vi "ExpDetailsHeader.vi"(0 "error in (no error)":errorcluster) -> (1 "appended array":string[][](array[string]), 2 "error out":errorcluster)   [LabVIEW 2020]
panel:
  in  "OK Button":bool
  in  "Operator":string
  in  "Target's material":string
  in  "Experiment number":string
  in  "Target's width":string
  in  "Bean Diameter":string
  in  "Laser Power [W]":string
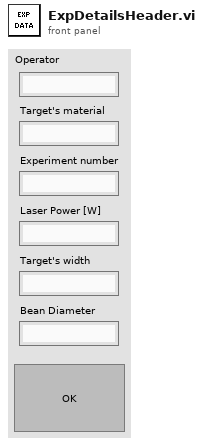
[diagram p1: front panel]
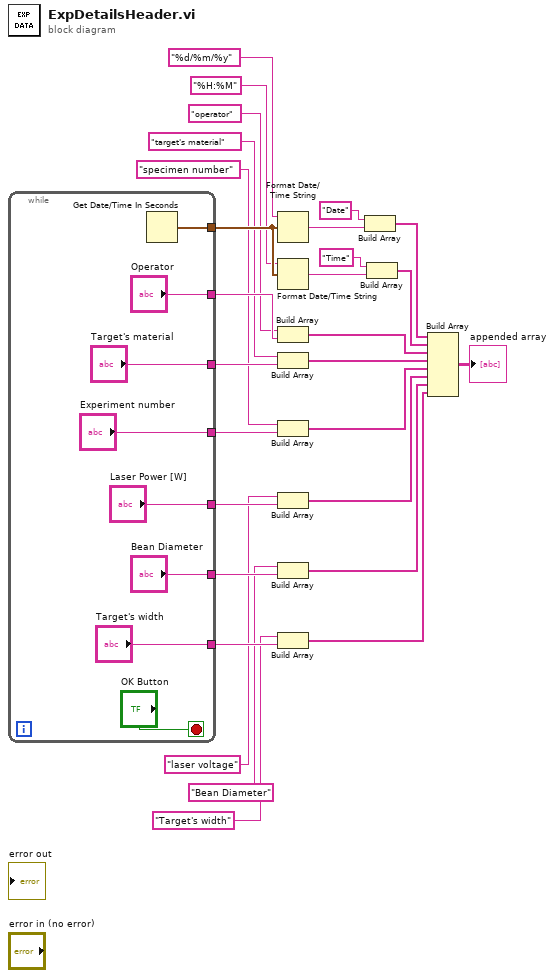
[diagram p0: block diagram]
diagram:
  n1 = while {
    tunnel: ["Laser Power [W]"] -> w28
    tunnel: ["Bean Diameter"] -> w27
    tunnel: ["Target's width"] -> w26
    tunnel: ["Experiment number"] -> w25
    tunnel: ["Target's material"] -> w24
    tunnel: ["Operator"] -> w23
    tunnel: [w29] -> w14
    stop <- "OK Button" stop-if-true
    n2 = Get Date/Time In Seconds() -> (seconds since 1Jan1904=w29:timestamp)
  }
  n3 = Format Date/Time String(time format string (%c)="%d/%m/%y", seconds (now)=w14) -> (date/time string=w7:string)  [unwired: 1 in]
  n4 = Format Date/Time String(time format string (%c)="%H:%M", seconds (now)=w14) -> (date/time string=w2:string)  [unwired: 1 in]
  n5 = Build Array("operator", w23) -> (w22:string[])
  n6 = Build Array("target's material", w24) -> (w21:string[])
  n7 = Build Array("specimen number", w25) -> (w20:string[])
  n8 = Build Array("laser voltage", w28) -> (w19:string[])
  n9 = Build Array("Bean Diameter", w27) -> (w18:string[])
  n10 = Build Array("Target's width", w26) -> (w17:string[])
  n11 = Build Array("Date", w7) -> (w5:string[])
  n12 = Build Array("Time", w2) -> (w4:string[])
  n13 = Build Array(w5, w4, w22, w21, w20, w19, w18, w17) -> (→"appended array":string[][])
